vi "Read Defaults.vi"(3 "error in (no error)":errorcluster, 5 "appended path":path) -> (0 "error out":errorcluster, 1 "massUnits":string, 2 "lengthUnits":string)   [LabVIEW 2015]
uses:
  <vilib>/Utility/config.llb/Read Key (String).vi
  <vilib>/Utility/config.llb/NI_LVConfig.lvlib
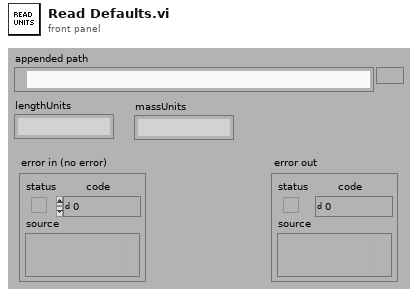
[diagram p1: front panel]
types:
  T1 = typedef "NI_LVConfig.lvlib/Config Data RefNum.ctl" = refnum<k1>
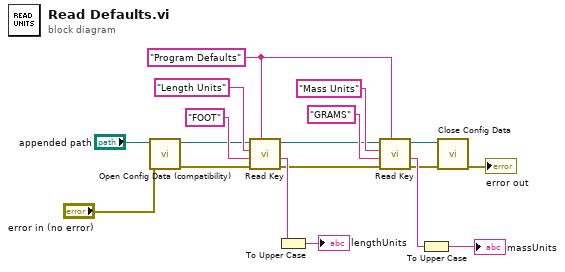
[diagram p0: block diagram]
diagram:
  w17 = "Program Defaults" ("section")
  n1 = call <vilib>:"Open Config Data (compatibility).vi"("error in (no error)"="error in (no error)", "configuration file path"="appended path") -> ("error out"=w14:errorcluster, "refnum"=w8:T1)  [unwired: 7 in, 1 out]
  n2 = call-poly <vilib>:"Read Key.vi"("section"=w17, "error in (no error)"=w14, "default value"="FOOT", "key"="Length Units", "refnum"=w8) -> ("error out"=w13:errorcluster, "value"=w16:string, "refnum out"=w11:T1)  [unwired: 1 in, 3 out]
  n3 = To Upper Case(1:w16) -> (0:→"lengthUnits":string)
  n4 = call-poly <vilib>:"Read Key.vi"("section"=w17, "error in (no error)"=w13, "default value"="GRAMS", "key"="Mass Units", "refnum"=w11) -> ("error out"=w3:errorcluster, "value"=w15:string, "refnum out"=w4:T1)  [unwired: 1 in, 3 out]
  n5 = To Upper Case(1:w15) -> (0:→"massUnits":string)
  n6 = call <vilib>:"Close Config Data.vi"("error in (no error)"=w3, "refnum"=w4) -> ("error out"=→"error out":errorcluster)  [unwired: 1 in, 8 out]
